vi "Set Menu Item Picture.vi"(7 "item tag":string, 8 "error in (no error)":errorcluster, 9 "Hilite Picture":refnum<class "Image.lvclass">, 10 "Picture":refnum<class "Image.lvclass">, 11 "Menu in":refnum<class "Menu.lvclass">) -> (0 "error out":errorcluster, 3 "Menu out":refnum<class "Menu.lvclass">)   [LabVIEW 2021, in "Menu.lvlib" / "Menu.lvclass"]
uses:
  Menu.lvclass
  Picture2D/src/Picture/Image.lvclass
  Picture2D/src/2DPictureControl/2DPictureControl.lvclass
  MenuItems.ctl
  <vilib>/Utility/miscctls.llb/LVMenuShortCut.ctl
  <vilib>/Utility/miscctls.llb/LVMapReplaceAction.ctl
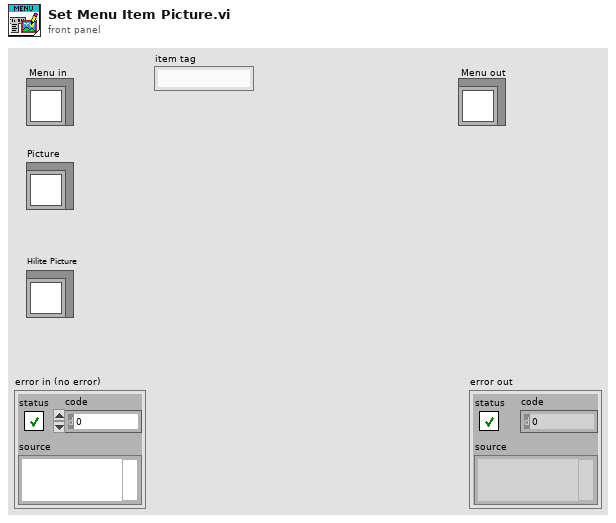
[diagram p1: front panel]
types:
  T1 = typedef "Menu.lvlib/Menu.lvclass/MenuItems.ctl" = cluster{"Item Name":string, "Short Cut":T2, "Checked":bool, "Enable":bool, "After item":string, "Item Tags":string[], "Item Names":string[], "Picture":refnum<class "Image.lvclass">, "Hilite Picture":refnum<class "Image.lvclass">, "Displayed":bool}
  T2 = typedef "LVMenuShortCut.ctl" = cluster{"Include Shift Key?":bool, "Include Ctrl Key?":bool, "Shortcut Key":string}
  T3 = typedef "LVMapReplaceAction.ctl" = enum32{"Modify Entry only if found", "Add or Modify Entry", "Delete Entry"}
  T4 = typedef "Menu.lvlib/Menu.lvclass/Data.ctl" = cluster{"MenuMap":map{string, T1}, "PictRef":refnum<vi>, "MenuSelectionEvent":refnum<user-event>, "TopMenuSpacing":i32, "MenuSpacing":i32, "CloseEvent":refnum<user-event>, "TR_ManageMenuRef":refnum<vi>, "MenuColors":T5, "RTMPath":path, "RTMVIReference":refnum<vi>, "RTMMenuReference":refnum<k9>, "CtlRef":refnum<vi>, "User-Specified Font":refnum<class "Font.lvclass">, "Desired Font":enum16{"User-specified Font", "Application Font", "System Font", "Dialog Font"}, "SubMenuIcon":T6, "SubMenuIconClosed":refnum<class "Picture2D.lvclass">, "SubMenuIconOpened":refnum<class "Picture2D.lvclass">}
  T5 = typedef "Menu.lvlib/Menu.lvclass/MenuColors.ctl" = cluster{"Text":refnum<class "Color.lvclass">, "HiliteText":refnum<class "Color.lvclass">, "Background":refnum<class "Color.lvclass">, "BorderColor":refnum<class "Color.lvclass">, "Hilite":refnum<class "Color.lvclass">}
  T6 = typedef "Menu.lvlib/Menu.lvclass/SubMenuIcon.ctl" = enum16{"LabVIEW", "Windows", "Custom"}
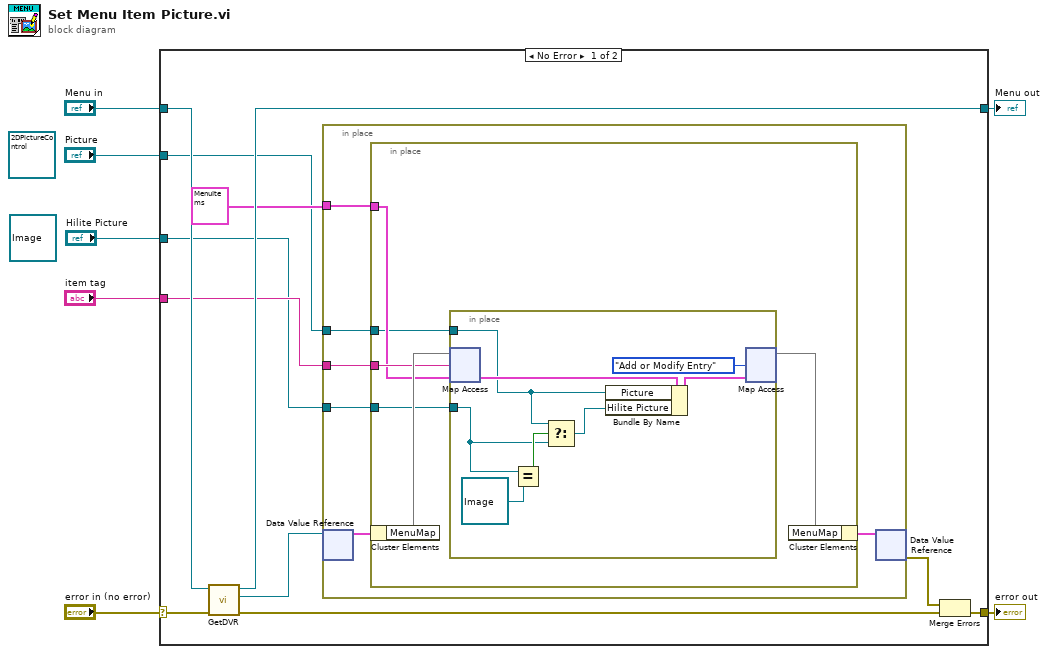
[diagram p0: block diagram]
diagram:
  (unwired) refnum<class "Image.lvclass"> refnum ("Hilite Picture")
  (unwired) refnum<class "2DPictureControl.lvclass"> refnum ("Picture")
  (unwired) refnum<class "2DPictureControl.lvclass"> refnum ("Picture")
  n1 = case shown="No Error" "error in (no error)" {
    selector: "error in (no error)" -> [w18 w40]
    tunnel: [w10 w40] -> w6
    tunnel: [w16 w39] -> w4
    tunnel: "Menu in" -> [w15 w39]
    tunnel: "item tag" -> [w13 _]
    tunnel: "Picture" -> [w11 _]
    tunnel: "Hilite Picture" -> [w8 _]
    frame No Error {
      n2 = call "GetDVR.vi"("error in (no error)"=w18, "Menu in"=w15) -> ("error out"=w17:errorcluster, "DVR"=w14:refnum<data-value>, "Menu out"=w16:refnum<class "Menu.lvclass">)  [unwired: 7 in]
      n3 = in-place {
        in-place-border: w13 -> [w23]
        in-place-border: T1 {"Item Name"="", "Short Cut"={"Include Shift Key?"=FALSE, "Include Ctrl Key?"=FALSE, "Shortcut Key"=""}, "Checked"=FALSE, "Enable"=FALSE, "After item"="", "Item Tags"=[], "Item Names"=[], "Picture"=refnum, "Hilite Picture"=refnum, "Displayed"=FALSE} ("Menu") -> [w21]
        in-place-border: w11 -> [w20]
        in-place-border: w8 -> [w19]
        n4 = in-place-dvr #1(w14) -> (w24:T4)  [unwired: 1 out]
        n5 = in-place {
          in-place-border: w23 -> [w29]
          in-place-border: w21 -> [w27]
          in-place-border: w20 -> [w26]
          in-place-border: w19 -> [w25]
          n6 = in-place-cluster #2(w24) -> ("MenuMap"=w30:map{string, T1})
          n7 = in-place {
            in-place-border: w26 -> [w34]
            in-place-border: w25 -> [w31]
            n8 = in-place-map #3(w30, w29, w27) -> (w37:T1)  [unwired: 1 out]
            n9 = Equal?(x=w31, y=refnum<class "Image.lvclass"> refnum ("Hilite Picture")) -> (x = y?=w33:bool)
            n10 = Select(t=w34, s=w33, f=w31) -> (s? t:f=w35:refnum<class "Image.lvclass">)
            n11 = Bundle By Name(cluster=w37, "Picture"=w34, "Hilite Picture"=w35) -> (w36:T1)
            n12 = in-place-map #3(w36, LVMapReplaceAction."Add or Modify Entry" ("action")) -> (w28:map{string, T1})  [unwired: 2 out]
          }
          n13 = in-place-cluster #2("MenuMap"=w28) -> (w22:T4)
        }
        n14 = in-place-dvr #1(w22) -> (w9:errorcluster)  [unwired: 1 out]
      }
      n15 = Merge Errors(w9, w17) -> (w10:errorcluster)
    }
    frame Error {
    }
  }
  "error out" <- w6
  "Menu out" <- w4
